vi "LD Control.vi"() -> ()   [LabVIEW 2017]
uses:
  <vilib>/Utility/error.llb/Clear Errors.vi
  <instrlib>/tio-labview/TIO Library/TIO RPC Send REQuest.vi
  <instrlib>/tio-labview/TIO Library/TIO RPC Parse Reply.vi
  <instrlib>/tio-labview/TIO Library/TIO RPC Parse Reply Error.vi
  <instrlib>/tio-labview/TIO Library/TIO Data Stream Parse timebase Info.vi
  <instrlib>/tio-labview/TIO Library/TIO Data Stream Parse pstream Info.vi
  <instrlib>/tio-labview/TIO Library/TIO Data Stream Parse dstream Info.vi
  <instrlib>/tio-labview/TIO Library/TIO Stream Write.vi
  <instrlib>/tio-labview/TIO Library/TIO RPC Form Request.vi
  <instrlib>/tio-labview/TIO Library/TIO SLIP Serial Write.vi
  <instrlib>/tio-labview/TIO Library/TIO Form Packet.vi
  <instrlib>/tio-labview/TIO Library/TIO SLIP Encode.vi
  <instrlib>/tio-labview/TIO Library/TIO Serial Checksum CRC32.vi
  <instrlib>/tio-labview/TIO Library/TIO Stream Read Non-blocking.vi
panel:
  in  "Current Enable":bool
  out "TEC Current Mon":dbl[unit] format="%#.3f"
  out "Laser Current Mon":dbl[unit] format="%#_4g"
  in  "Cal Temperature":dbl[unit] format="%#_4g"
  in  "Laser Current Max":dbl[unit] format="%#_4g"
  in  "Laser Current":dbl[unit] format="%#_4g"
  in  "Manual Current":bool
  in  "Autostart":bool
  in  "Ki":dbl format="%#_4g"
  in  "Kp":dbl format="%#_4g"
  out "Resistance":dbl[unit] format="%#_4g"
  in  "Save":bool
  in  "Calibrate R0":bool
  in  "TEC Enable":bool
  out "TEC Current":dbl[unit] format="%#_4f"
  in  "TEC Current Max":dbl[unit] format="%#_4f"
  out "Temperature":dbl[unit] format="%#_4g"
  in  "Temperature Set":dbl[unit] format="%#_4g"
  in  "URL":refnum<visa-resource-name>="tcp://localhost"
  out "ID":string
  in  "Quit":bool
  in  "Duration":dbl[unit]=100.0
  in  "Reset":bool
  out "Laser Current Graph":T1(graph)
  out "Temperature Graph":T1(graph)
  out "TEC Current Graph":T1(graph)
  # "Laser Driver"
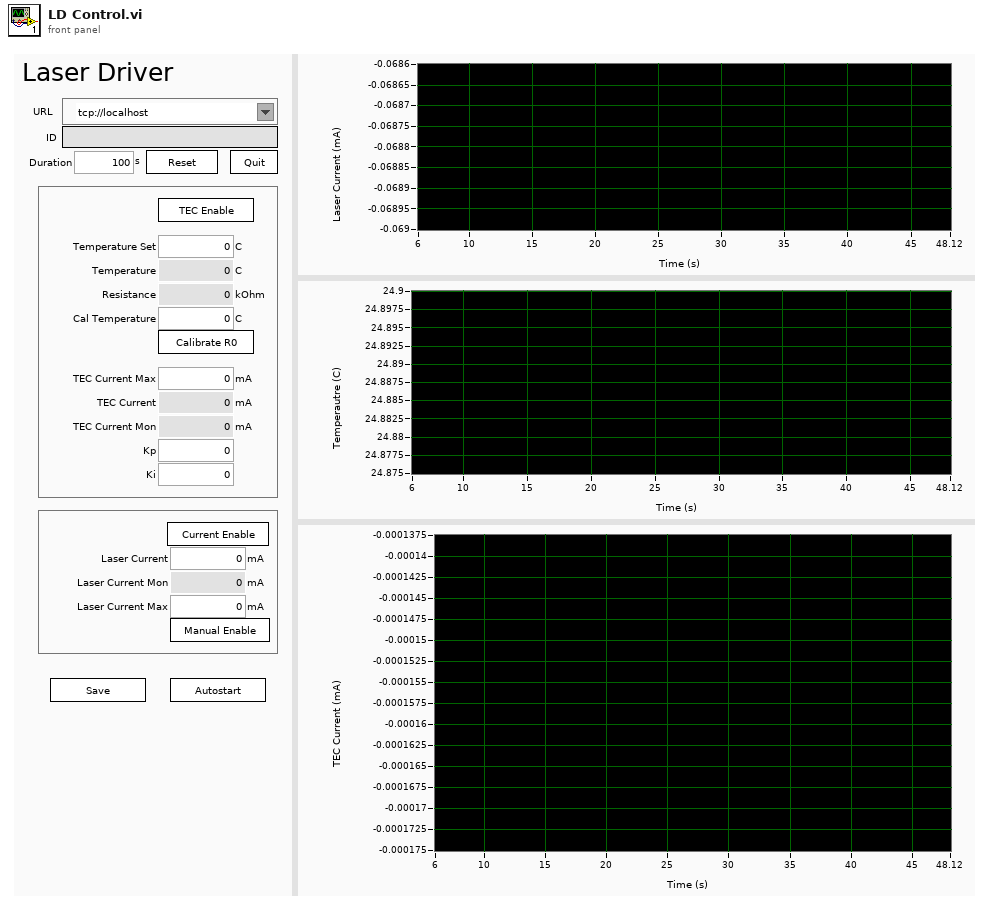
[diagram p1: front panel]
types:
  T1 = cluster{"start":dbl, "dt":dbl, "Timeseries":dbl[]}
  T2 = cluster{"TS Connection":cluster{"Type":enum16{"TCP", "Serial"}, "URL":refnum<visa-resource-name>, "TCP":refnum<k5>, "Timeout":u32, "Route":string}, "REQ":refnum<queue>, "REP":refnum<queue>}
  T3 = cluster{"Awaiting REP":bool, "REQ ID":u32, "dstreams in":cluster{"id":u16, "timebase id":u16, "period":u32, "offset":u32, "sample number":u64, "total components":u16, "flags":u16, "components":cluster{"pstream id":u16, "flags":u16, "period":u32, "offset":u32}[]}[], "pstreams":cluster{"id":u16, "timebase_id":u16, "period":u32, "offset":u32, "fmt":i32, "flags":u16, "channels":u16, "type":u8, "name":string, "column names":string[], "title":string, "units":string}[], "timebases":cluster{"id":u16, "source":u16, "epoch":u32, "start time":u32, "period numerator (µs)":i32, "period denominator (µs)":u16, "flags":u16, "stability":u8, "source id":string}[]}
  T4 = cluster{"dstream ID":u16, "Sample Number":u32, "Raw Data":string}
  T5 = cluster{"Name":string, "Waveform":cluster{"start":dbl, "dt":dbl, "Timeseries":dbl[][]}}[]
  T6 = cluster{"start":dbl, "dt":dbl, "Timeseries":dbl[][]}
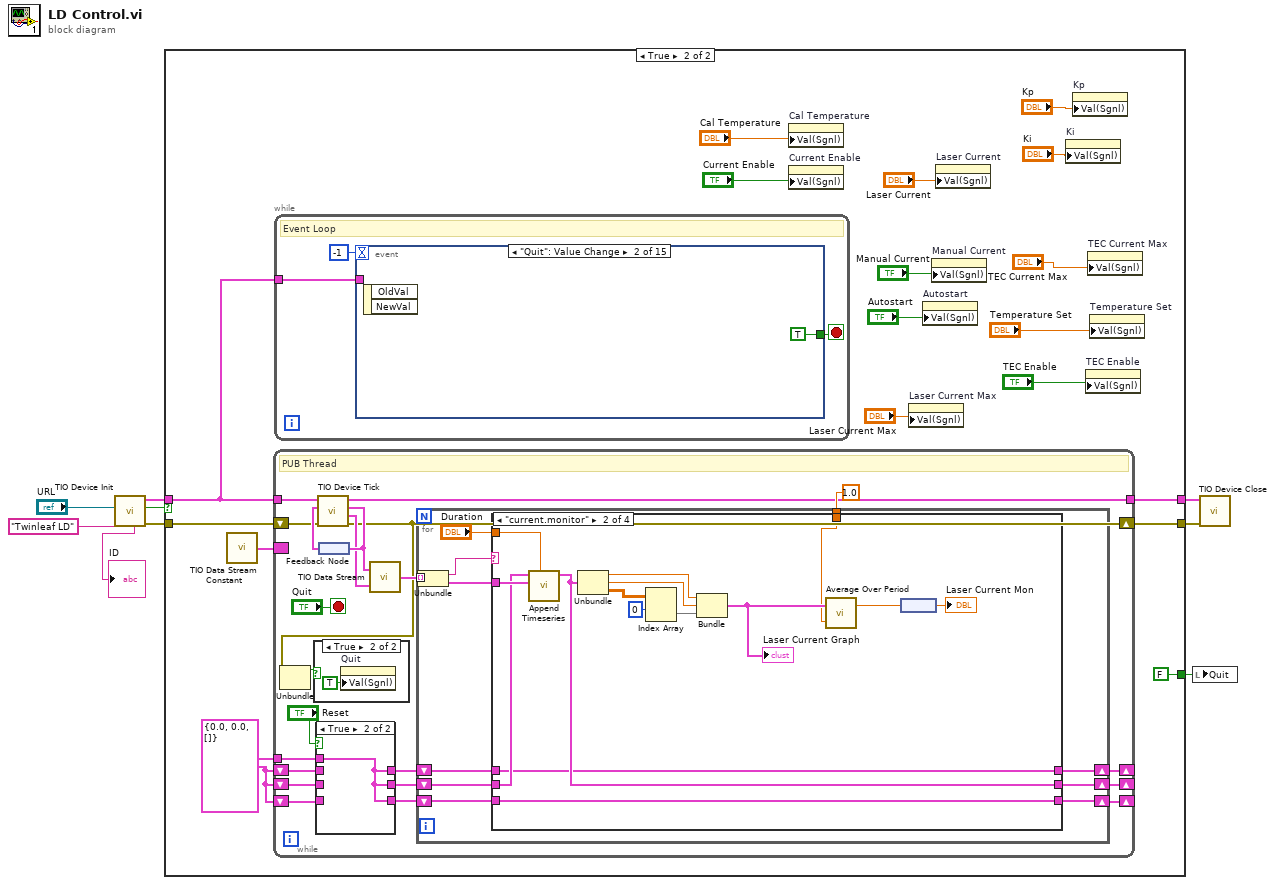
[diagram p0: block diagram]
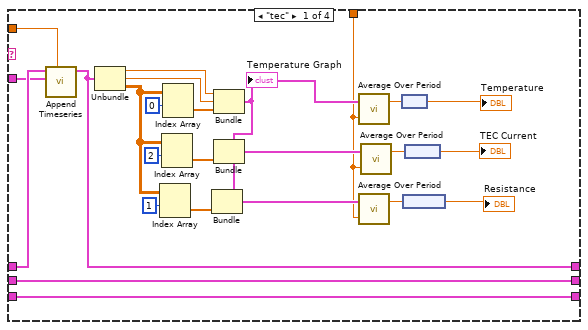
[diagram p5: hidden frame]
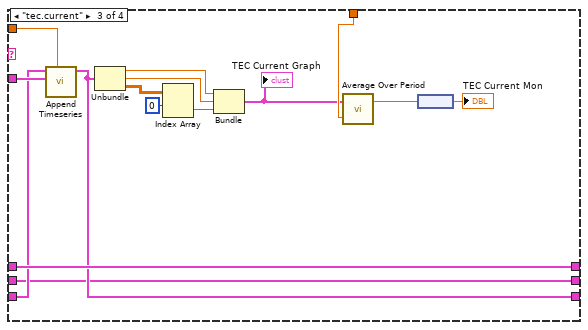
[diagram p6: hidden frame]
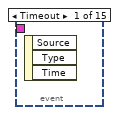
[diagram p8: hidden frame]
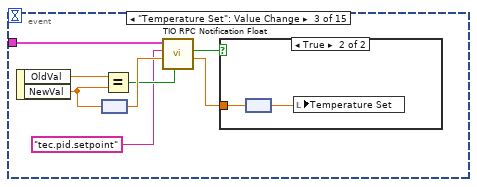
[diagram p9: hidden frame]
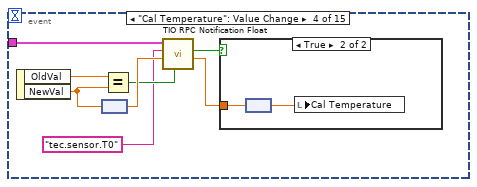
[diagram p11: hidden frame]
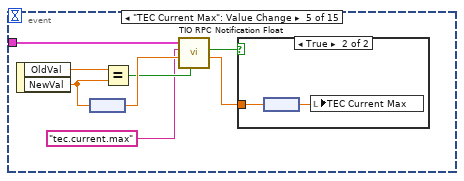
[diagram p13: hidden frame]
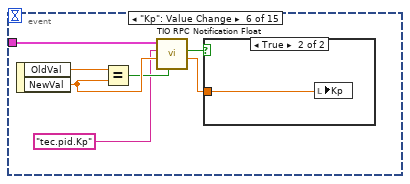
[diagram p15: hidden frame]
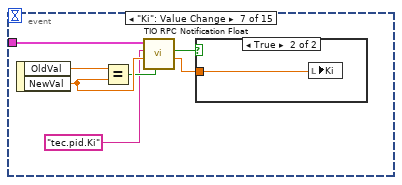
[diagram p17: hidden frame]
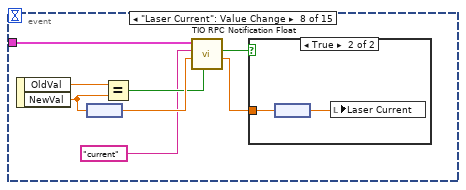
[diagram p19: hidden frame]
diagram:
  n1 = call <instrlib>:"TIO Device Init.vi"("ID"="Twinleaf LD", "URL"="URL") -> ("error out"=w5:errorcluster, 2:"ID Verified"=w6:bool, "TIO"=w7:T2, 4:"ID Verified"=→"ID":string)  [unwired: 5 in, 1 out]
  n2 = case shown="True" w6 {
    tunnel: w7 -> [w11 w18]
    tunnel: w5 -> [w10 w19]
    tunnel: [_ FALSE ("Quit")] -> w4
    tunnel: [w10 w13] -> w3
    tunnel: [w11 w12] -> w2
    frame False {
    }
    frame True {
      w15 = cluster{dbl, dbl, dbl[][]} {0.0, 0.0, []} ("Waveform Timeseries")
      n3 = call <instrlib>:"TIO Data Stream Constant.vi"() -> ("TIO State"=w20:T3)
      n4 = while {
        shift-right: [w51] -> _
        shift-left: w15 -> [w41]
        border: w20 -> [_]
        tunnel: w18 -> [w47]
        tunnel: w15 -> [w40]
        shift-right: [w38] -> _
        shift-left: w15 -> [w37]
        shift-right: [w34] -> _
        shift-left: w15 -> [w35]
        tunnel: [w31] -> w12
        shift-right: [w30] -> w13
        shift-left: w19 -> [w46]
        stop <- "Quit" stop-if-true
        # "PUB Thread"
        n5 = case shown="True" "Reset" {
          tunnel: [w55 w56] -> w42
          tunnel: w41 -> [w55 _]
          tunnel: w40 -> [_ w56]
          tunnel: [w54 w56] -> w39
          tunnel: w37 -> [w54 _]
          tunnel: w35 -> [w53 _]
          tunnel: [w53 w56] -> w36
          frame False {
          }
          frame True {
          }
        }
        n6 = feedback #1() -> (w50:T3)
        n7 = call <instrlib>:"TIO Device Tick.vi"("Error in"=w46, "TIO State"=w50, "TIO"=w47) -> ("Error out"=w30:errorcluster, "Data Out"=w48:T4, "TIO State"=w49:T3, "TIO Out"=w31:T2)  [unwired: 5 in]
        n8 = Unbundle(w30) -> ("status"=w32:bool)  [unwired: 2 out]
        n9 = case shown="True" w32 {
          frame False {
          }
          frame True {
            n10 = property on="Quit" class="Bool (strict)"("Val(Sgnl)"=TRUE ("Value (Signaling)")) -> ()  [unwired: 2 in, 2 out]
          }
        }
        n11 = feedback-in #1(w49) -> ()
        n12 = call <instrlib>:"TIO Data Stream.vi"("Raw Data"=w48, "TIO State"=w49) -> ("Data Out"=w45:T5)
        n13 = for {
          shift-right: [w66] -> w51
          shift-left: w42 -> [w65]
          tunnel: w45 -> [w64] mode=indexing
          shift-right: [w60] -> w38
          shift-left: w39 -> [w61]
          shift-right: [w58] -> w34
          shift-left: w36 -> [w59]
          tunnel: dbl[unit] 1.0 ("Period") -> [w57]
          n14 = Unbundle(w64) -> ("Name"=w62:string, "Waveform"=w63:T6)
          n15 = case shown="\"current.monitor\"" w62 {
            tunnel: "Duration" -> [w92 w107 w122 _]
            tunnel: [w90 w95 w114 w125] -> w66
            tunnel: w65 -> [w89 w95 w114 w125]
            tunnel: w63 -> [w71 w100 w115 _]
            tunnel: w61 -> [w70 w97 w108 w124]
            tunnel: [w70 w96 w108 w124] -> w60
            tunnel: [w69 w98 w109 w123] -> w58
            tunnel: w59 -> [w69 w98 w110 w123]
            tunnel: w57 -> [w68 w93 w112 _]
            frame "tec" {
              n16 = call <instrlib>:"Append Timeseries.vi"("Duration"=w92, "In New"=w71, "In Old"=w89) -> ("Appended"=w90:T6)  [unwired: 8 in]
              n17 = Unbundle(w90) -> ("start"=w75:dbl, "dt"=w74:dbl, "Timeseries"=w76:dbl[][])
              n18 = Index Array(array=w76, index (row)=1 ("disabled index (col)")) -> (element=w78:dbl[])  [unwired: 1 in]
              n19 = Index Array(array=w76, index (row)=2 ("disabled index (col)")) -> (element=w84:dbl[])  [unwired: 1 in]
              n20 = Index Array(array=w76, index (row)=0 ("disabled index (col)")) -> (element=w88:dbl[])  [unwired: 1 in]
              n21 = Bundle("start"=w75, "dt"=w74, "Timeseries"=w88) -> (w72:T1)  [unwired: 1 in]
              "Temperature Graph" <- w72
              n22 = Bundle(cluster=w72, "Timeseries"=w78) -> (w79:T1)  [unwired: 2 in]
              n23 = Bundle(cluster=w72, "Timeseries"=w84) -> (w83:T1)  [unwired: 2 in]
              n24 = call <instrlib>:"Average Over Period.vi"("Period"=w68, "Cluster"=w72) -> ("Average"=w87:dbl)  [unwired: 1 in]
              n25 = call <instrlib>:"Average Over Period.vi"("Period"=w68, "Cluster"=w79) -> ("Average"=w80:dbl)  [unwired: 1 in]
              n26 = call <instrlib>:"Average Over Period.vi"("Period"=w68, "Cluster"=w83) -> ("Average"=w82:dbl)  [unwired: 1 in]
              n27 = node(w87) -> (→"Temperature":dbl[unit])
              n28 = node(w80) -> (→"Resistance":dbl[unit])
              n29 = node(w82) -> (→"TEC Current":dbl[unit])
            }
            frame "current.monitor" {
              n30 = call <instrlib>:"Append Timeseries.vi"("Duration"=w107, "In New"=w100, "In Old"=w97) -> ("Appended"=w96:T6)  [unwired: 8 in]
              n31 = Unbundle(w96) -> ("start"=w102:dbl, "dt"=w101:dbl, "Timeseries"=w103:dbl[][])
              n32 = Index Array(array=w103, index (row)=0 ("disabled index (col)")) -> (element=w105:dbl[])  [unwired: 1 in]
              n33 = Bundle("start"=w102, "dt"=w101, "Timeseries"=w105) -> (w99:T1)  [unwired: 1 in]
              "Laser Current Graph" <- w99
              n34 = call <instrlib>:"Average Over Period.vi"("Period"=w93, "Cluster"=w99) -> ("Average"=w104:dbl)  [unwired: 1 in]
              n35 = node(w104) -> (→"Laser Current Mon":dbl[unit])
            }
            frame "tec.current" {
              n36 = call <instrlib>:"Append Timeseries.vi"("Duration"=w122, "In New"=w115, "In Old"=w110) -> ("Appended"=w109:T6)  [unwired: 8 in]
              n37 = Unbundle(w109) -> ("start"=w117:dbl, "dt"=w116:dbl, "Timeseries"=w118:dbl[][])
              n38 = Index Array(array=w118, index (row)=0 ("disabled index (col)")) -> (element=w120:dbl[])  [unwired: 1 in]
              n39 = Bundle("start"=w117, "dt"=w116, "Timeseries"=w120) -> (w111:T1)  [unwired: 1 in]
              "TEC Current Graph" <- w111
              n40 = call <instrlib>:"Average Over Period.vi"("Period"=w112, "Cluster"=w111) -> ("Average"=w119:dbl)  [unwired: 1 in]
              n41 = node(w119) -> (→"TEC Current Mon":dbl[unit])
            }
            frame Default {
            }
          }
        }
      }
      n42 = while {
        tunnel: w18 -> [w127]
        stop <- w126 stop-if-true
        # "Event Loop"
        n43 = event shown="[1] \"Quit\": Value Change" {
          selector: _ -> [_ _ _ _ _ _ _ _ _ _ _ _ _ _ _]
          dyn-events: _ -> [_ _ _ _ _ _ _ _ _ _ _ _ _ _ _]
          timeout: -1 -> [_ _ _ _ _ _ _ _ _ _ _ _ _ _ _]
          tunnel: w127 -> [_ _ w132 w142 w152 w162 w169 w178 w188 w198 w208 w218 w229 w239 w241]
          tunnel: [_ TRUE ("Quit") _ _ _ _ _ _ _ _ _ _ _ _ _] -> w126
          event Timeout {
            n44 = event-data() -> ()  [unwired: 1 in, 3 out]
          }
          event "Quit": Value Change {
            n45 = event-data() -> ()  [unwired: 1 in, 2 out]
          }
          event "Temperature Set": Value Change {
            n46 = event-data() -> ("OldVal"=w137:dbl[unit], "NewVal"=w133:dbl[unit])  [unwired: 1 in]
            n47 = node(w133) -> (w136:dbl)
            n48 = Equal?(x=w137, y=w133) -> (x = y?=w131:bool)
            n49 = call <instrlib>:"TIO RPC Notification Float.vi"("Read"=w131, "Set value"=w136, "Topic"="tec.pid.setpoint" ("String"), "TIO"=w132) -> ("Get value (default if error)"=w134:sgl, "Response"=w135:bool)  [unwired: 4 in, 1 out]
            n50 = case shown="True" w135 {
              tunnel: w134 -> [_ w139]
              frame False {
              }
              frame True {
                n51 = node(w139) -> (w138:sgl[unit])
                n52 = local write "Temperature Set"(w138) -> ()
              }
            }
          }
          event "Cal Temperature": Value Change {
            n53 = event-data() -> ("OldVal"=w147:dbl[unit], "NewVal"=w143:dbl[unit])  [unwired: 1 in]
            n54 = node(w143) -> (w146:dbl)
            n55 = Equal?(x=w147, y=w143) -> (x = y?=w141:bool)
            n56 = call <instrlib>:"TIO RPC Notification Float.vi"("Read"=w141, "Set value"=w146, "Topic"="tec.sensor.T0" ("String"), "TIO"=w142) -> ("Get value (default if error)"=w144:sgl, "Response"=w145:bool)  [unwired: 4 in, 1 out]
            n57 = case shown="True" w145 {
              tunnel: w144 -> [_ w149]
              frame False {
              }
              frame True {
                n58 = node(w149) -> (w148:sgl[unit])
                n59 = local write "Cal Temperature"(w148) -> ()
              }
            }
          }
          event "TEC Current Max": Value Change {
            n60 = event-data() -> ("OldVal"=w157:dbl[unit], "NewVal"=w153:dbl[unit])  [unwired: 1 in]
            n61 = node(w153) -> (w156:dbl)
            n62 = Equal?(x=w157, y=w153) -> (x = y?=w151:bool)
            n63 = call <instrlib>:"TIO RPC Notification Float.vi"("Read"=w151, "Set value"=w156, "Topic"="tec.current.max" ("String"), "TIO"=w152) -> ("Get value (default if error)"=w154:sgl, "Response"=w155:bool)  [unwired: 4 in, 1 out]
            n64 = case shown="True" w155 {
              tunnel: w154 -> [_ w159]
              frame False {
              }
              frame True {
                n65 = node(w159) -> (w158:sgl[unit])
                n66 = local write "TEC Current Max"(w158) -> ()
              }
            }
          }
          event "Kp": Value Change {
            n67 = event-data() -> ("OldVal"=w166:dbl, "NewVal"=w163:dbl)  [unwired: 1 in]
            n68 = Equal?(x=w166, y=w163) -> (x = y?=w161:bool)
            n69 = call <instrlib>:"TIO RPC Notification Float.vi"("Read"=w161, "Set value"=w163, "Topic"="tec.pid.Kp" ("String"), "TIO"=w162) -> ("Get value (default if error)"=w164:sgl, "Response"=w165:bool)  [unwired: 4 in, 1 out]
            n70 = case shown="True" w165 {
              tunnel: w164 -> [_ w167]
              frame False {
              }
              frame True {
                n71 = local write "Kp"(w167) -> ()
              }
            }
          }
          event "Ki": Value Change {
            n72 = event-data() -> ("OldVal"=w174:dbl, "NewVal"=w171:dbl)  [unwired: 1 in]
            n73 = Equal?(x=w174, y=w171) -> (x = y?=w170:bool)
            n74 = call <instrlib>:"TIO RPC Notification Float.vi"("Read"=w170, "Set value"=w171, "Topic"="tec.pid.Ki" ("String"), "TIO"=w169) -> ("Get value (default if error)"=w172:sgl, "Response"=w173:bool)  [unwired: 4 in, 1 out]
            n75 = case shown="True" w173 {
              tunnel: w172 -> [_ w175]
              frame False {
              }
              frame True {
                n76 = local write "Ki"(w175) -> ()
              }
            }
          }
          event "Laser Current": Value Change {
            n77 = event-data() -> ("OldVal"=w183:dbl[unit], "NewVal"=w179:dbl[unit])  [unwired: 1 in]
            n78 = node(w179) -> (w182:dbl)
            n79 = Equal?(x=w183, y=w179) -> (x = y?=w177:bool)
            n80 = call <instrlib>:"TIO RPC Notification Float.vi"("Read"=w177, "Set value"=w182, "Topic"="current" ("String"), "TIO"=w178) -> ("Get value (default if error)"=w180:sgl, "Response"=w181:bool)  [unwired: 4 in, 1 out]
            n81 = case shown="True" w181 {
              tunnel: w180 -> [_ w185]
              frame False {
              }
              frame True {
                n82 = node(w185) -> (w184:sgl[unit])
                n83 = local write "Laser Current"(w184) -> ()
              }
            }
          }
          event "Laser Current Max": Value Change {
            n84 = event-data() -> ("OldVal"=w193:dbl[unit], "NewVal"=w189:dbl[unit])  [unwired: 1 in]
            n85 = node(w189) -> (w192:dbl)
            n86 = Equal?(x=w193, y=w189) -> (x = y?=w187:bool)
            n87 = call <instrlib>:"TIO RPC Notification Float.vi"("Read"=w187, "Set value"=w192, "Topic"="current.max" ("String"), "TIO"=w188) -> ("Get value (default if error)"=w190:sgl, "Response"=w191:bool)  [unwired: 4 in, 1 out]
            n88 = case shown="True" w191 {
              tunnel: w190 -> [_ w195]
              frame False {
              }
              frame True {
                n89 = node(w195) -> (w194:sgl[unit])
                n90 = local write "Laser Current Max"(w194) -> ()
              }
            }
          }
          event "TEC Enable": Value Change {
            n91 = event-data() -> ("OldVal"=w203:bool, "NewVal"=w199:bool)  [unwired: 1 in]
            n92 = Equal?(x=w203, y=w199) -> (x = y?=w197:bool)
            n93 = Boolean To (0,1)(Boolean=w199) -> (0, 1=w202:i16)
            n94 = call <instrlib>:"TIO RPC Notification U8.vi"("Read"=w197, "U8"=w202, "Topic"="tec.enable" ("String"), "TIO"=w198) -> ("U8"=w200:u8, "Response"=w201:bool)  [unwired: 4 in, 1 out]
            n95 = case shown="True" w201 {
              tunnel: w200 -> [_ w205]
              frame False {
              }
              frame True {
                n96 = Greater Than 0?(x=w205) -> (x > 0?=w204:bool)
                n97 = local write "TEC Enable"(w204) -> ()
              }
            }
          }
          event "Current Enable": Value Change {
            n98 = event-data() -> ("OldVal"=w213:bool, "NewVal"=w209:bool)  [unwired: 1 in]
            n99 = Equal?(x=w213, y=w209) -> (x = y?=w207:bool)
            n100 = Boolean To (0,1)(Boolean=w209) -> (0, 1=w212:i16)
            n101 = call <instrlib>:"TIO RPC Notification U8.vi"("Read"=w207, "U8"=w212, "Topic"="current.enable" ("String"), "TIO"=w208) -> ("U8"=w210:u8, "Response"=w211:bool)  [unwired: 4 in, 1 out]
            n102 = case shown="True" w211 {
              tunnel: w210 -> [_ w215]
              frame False {
              }
              frame True {
                n103 = Greater Than 0?(x=w215) -> (x > 0?=w214:bool)
                n104 = local write "Current Enable"(w214) -> ()
              }
            }
          }
          event "Autostart": Value Change {
            n105 = event-data() -> ("OldVal"=w223:bool, "NewVal"=w219:bool)  [unwired: 1 in]
            n106 = Equal?(x=w223, y=w219) -> (x = y?=w217:bool)
            n107 = Boolean To (0,1)(Boolean=w219) -> (0, 1=w222:i16)
            n108 = call <instrlib>:"TIO RPC Notification U8.vi"("Read"=w217, "U8"=w222, "Topic"="laser.autostart" ("String"), "TIO"=w218) -> ("U8"=w220:u8, "Response"=w221:bool)  [unwired: 4 in, 1 out]
            n109 = case shown="True" w221 {
              tunnel: w220 -> [_ w225]
              frame False {
              }
              frame True {
                n110 = Greater Than 0?(x=w225) -> (x > 0?=w224:bool)
                n111 = local write "Autostart"(w224) -> ()
              }
            }
          }
          event "Manual Current": Value Change {
            n112 = event-data() -> ("OldVal"=w234:bool, "NewVal"=w227:bool)  [unwired: 1 in]
            n113 = Equal?(x=w234, y=w227) -> (x = y?=w230:bool)
            n114 = Not(x=w227) -> (.not. x?=w226:bool)
            n115 = Boolean To (0,1)(Boolean=w226) -> (0, 1=w233:i16)
            n116 = call <instrlib>:"TIO RPC Notification U8.vi"("Read"=w230, "U8"=w233, "Topic"="laser.tecinterlock" ("String"), "TIO"=w229) -> ("U8"=w231:u8, "Response"=w232:bool)  [unwired: 4 in, 1 out]
            n117 = case shown="True" w232 {
              tunnel: w231 -> [_ w237]
              frame False {
              }
              frame True {
                n118 = Greater Than 0?(x=w237) -> (x > 0?=w236:bool)
                n119 = Not(x=w236) -> (.not. x?=w235:bool)
                n120 = local write "Manual Current"(w235) -> ()
              }
            }
          }
          event "Calibrate R0": Value Change {
            n121 = event-data() -> ()  [unwired: 1 in, 2 out]
            n122 = call <instrlib>:"TIO RPC Notification.vi"("Topic"="tec.sensor.R0.capture" ("String"), "TIO"=w239) -> ()  [unwired: 6 in, 3 out]
          }
          event "Save": Value Change {
            n123 = event-data() -> ()  [unwired: 1 in, 2 out]
            n124 = call <instrlib>:"TIO RPC Notification.vi"("Topic"="dev.conf.save" ("String"), "TIO"=w241) -> ()  [unwired: 6 in, 3 out]
          }
        }
      }
      n125 = property on="Cal Temperature" class="DigNum (strict)"("Val(Sgnl)"="Cal Temperature") -> ()  [unwired: 2 in, 2 out]
      n126 = property on="Current Enable" class="Bool (strict)"("Val(Sgnl)"="Current Enable") -> ()  [unwired: 2 in, 2 out]
      n127 = property on="Laser Current Max" class="DigNum (strict)"("Val(Sgnl)"="Laser Current Max") -> ()  [unwired: 2 in, 2 out]
      n128 = property on="Autostart" class="Bool (strict)"("Val(Sgnl)"="Autostart") -> ()  [unwired: 2 in, 2 out]
      n129 = property on="Manual Current" class="Bool (strict)"("Val(Sgnl)"="Manual Current") -> ()  [unwired: 2 in, 2 out]
      n130 = property on="Laser Current" class="DigNum (strict)"("Val(Sgnl)"="Laser Current") -> ()  [unwired: 2 in, 2 out]
      n131 = property on="Ki" class="DigNum (strict)"("Val(Sgnl)"="Ki") -> ()  [unwired: 2 in, 2 out]
      n132 = property on="Kp" class="DigNum (strict)"("Val(Sgnl)"="Kp") -> ()  [unwired: 2 in, 2 out]
      n133 = property on="TEC Enable" class="Bool (strict)"("Val(Sgnl)"="TEC Enable") -> ()  [unwired: 2 in, 2 out]
      n134 = property on="TEC Current Max" class="DigNum (strict)"("Val(Sgnl)"="TEC Current Max") -> ()  [unwired: 2 in, 2 out]
      n135 = property on="Temperature Set" class="DigNum (strict)"("Val(Sgnl)"="Temperature Set") -> ()  [unwired: 2 in, 2 out]
    }
  }
  n136 = local write "Quit"(w4) -> ()
  n137 = call <instrlib>:"TIO Device Close.vi"("Error in"=w3, "TIO"=w2) -> ()  [unwired: 10 in]
